vi "cic_test3.vi"() -> ()   [LabVIEW 2013]
panel:
  out "Waveform Graph out 2":i16[](graph)
  out "Waveform Graph out":dbl[](graph)
  out "Waveform Graph":dbl[](graph)
  out "# of Iterations":i32
  out "# of samples":i32
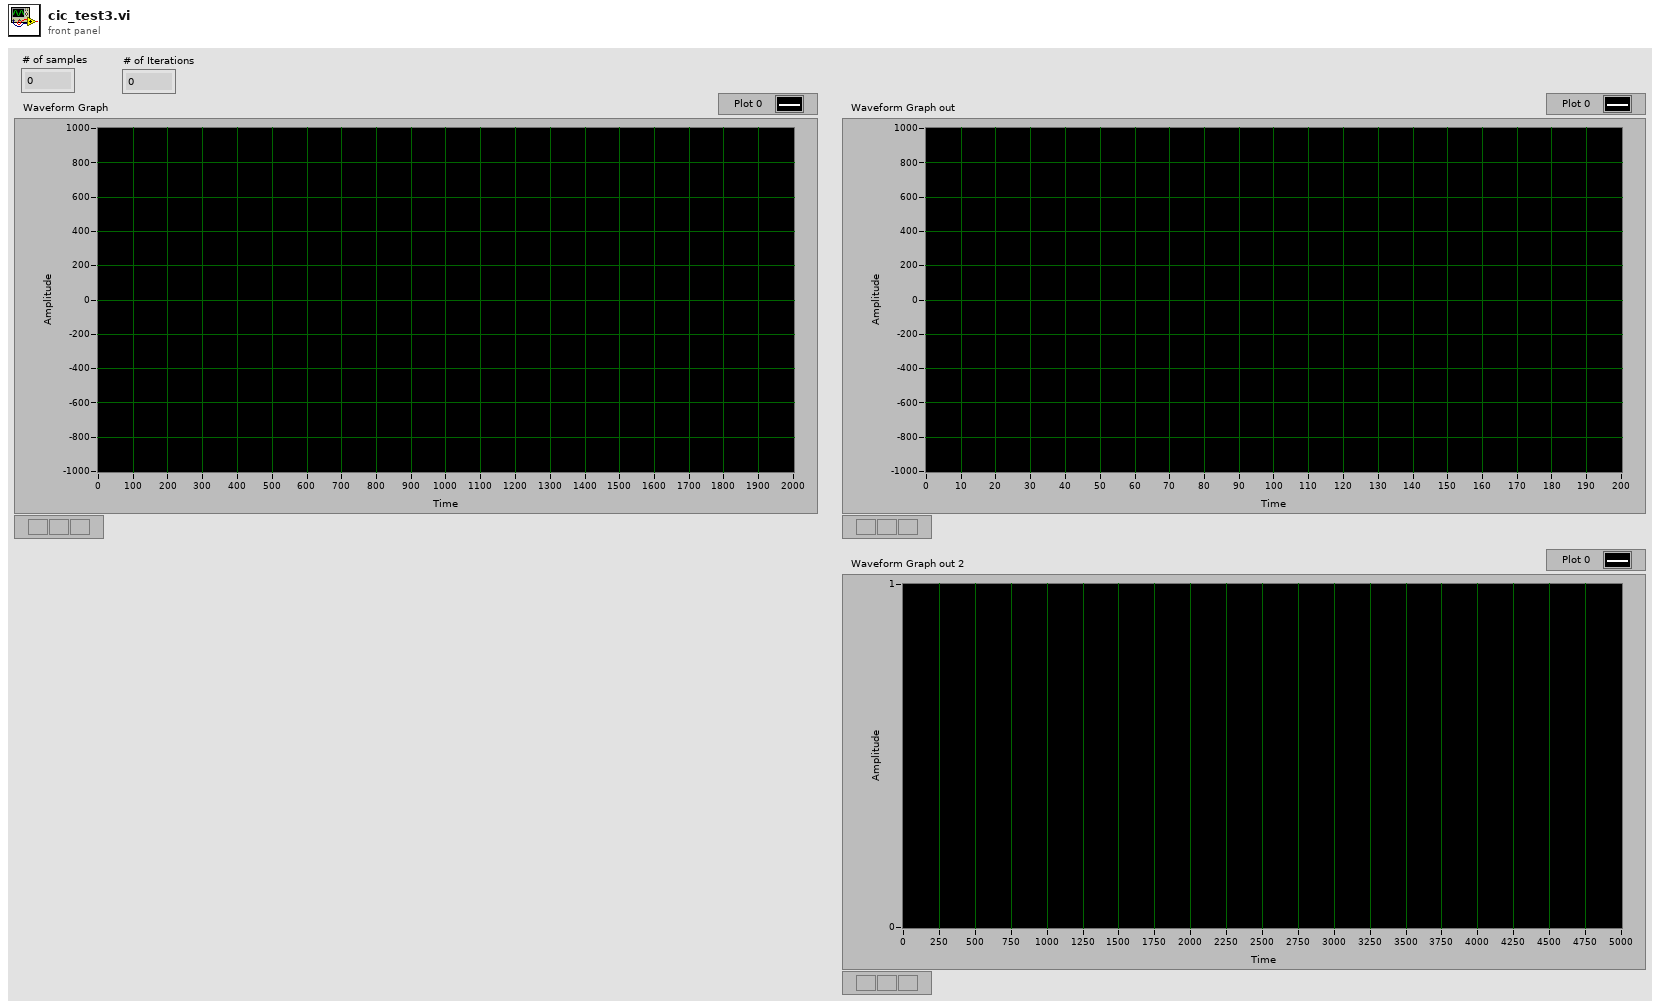
[diagram p1: front panel]
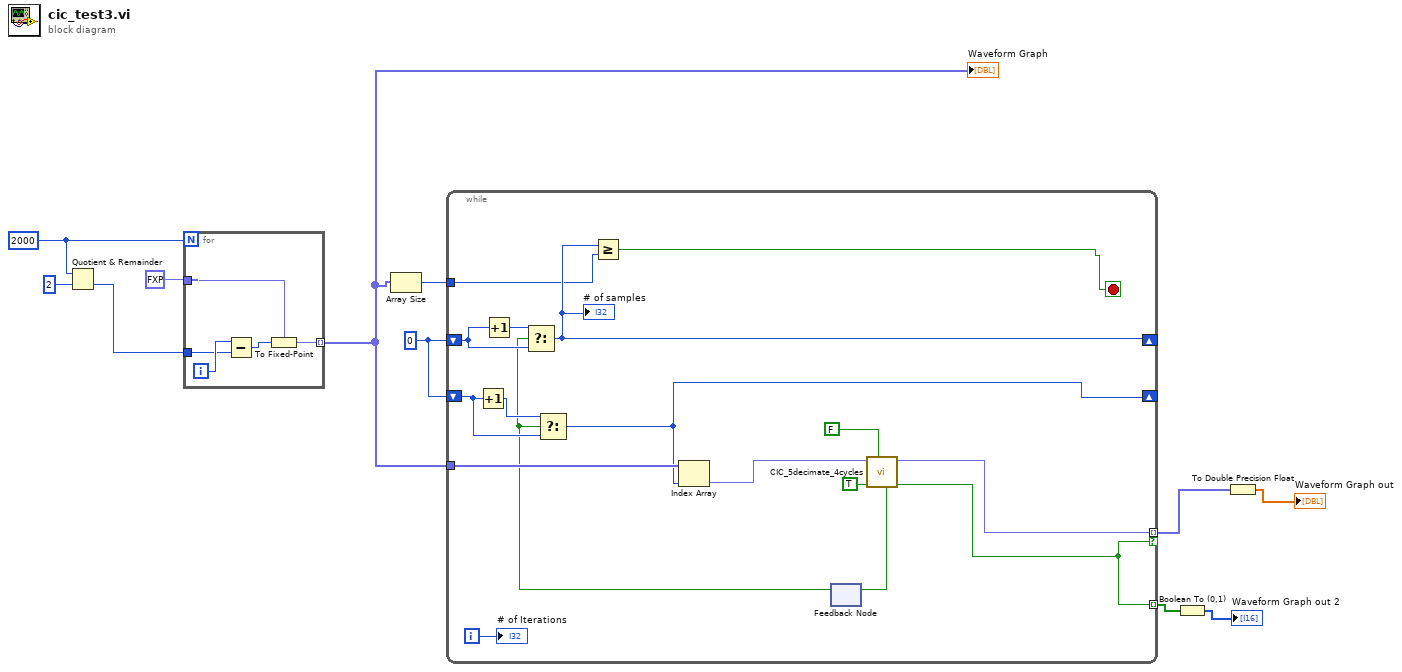
[diagram p0: block diagram]
diagram:
  w5 = 2000
  w9 = 0 ("samples")
  n1 = Quotient & Remainder(x=w5, y=2) -> (floor(x/y)=w3:i32)  [unwired: 1 out]
  n2 = for {
    N: w5 -> [_]
    tunnel: fxp<+/-,16,14> 0.0 ("fixed-point type") -> [w16]
    tunnel: [w15] -> w6 mode=indexing
    tunnel: w3 -> [w13]
    i -> [w14]
    n3 = Subtract(x=w14, y=w13) -> (x-y=w12:i32)
    n4 = To Fixed-Point(fixed-point type=w16, number=w12) -> (fixed-point=w15:fxp<+/-,16,14>)
  }
  "Waveform Graph" <- w6
  n5 = Array Size(array=w6) -> (size(s)=w10:i32)
  n6 = while {
    tunnel: w6 -> [w33]
    shift-right: [w25] -> _
    shift-left: w9 -> [w31]
    shift-right: [w28] -> _
    shift-left: w9 -> [w29]
    tunnel: [w19] -> w8 mode=indexing if=w17
    tunnel: w10 -> [w26]
    tunnel: [w17] -> w2 mode=indexing
    i -> [w24]
    stop <- w27 stop-if-true
    n7 = Increment(x=w31) -> (x+1=w32:i32)
    n8 = Increment(x=w29) -> (x+1=w30:i32)
    n9 = feedback #1() -> (w18:bool)  [unwired: 1 in]
    n10 = Select(t=w30, s=w18, f=w29) -> (s? t:f=w28:i32)
    "# of samples" <- w28
    n11 = Select(t=w32, s=w18, f=w31) -> (s? t:f=w25:i32)
    n12 = Greater Or Equal?(x=w28, y=w26) -> (x >= y?=w27:bool)
    n13 = Index Array(array=w33, index=w25) -> (element=w23:fxp<+/-,16,14>)
    n14 = call "CIC_5decimate_4cycles.vi"("reset"=FALSE, "valid in"=TRUE, "Data in"=w23) -> ("valid out"=w17:bool, "Data out"=w19:fxp<+/-,16,14>, "ready for input"=w22:bool)  [unwired: 6 in]
    n15 = feedback-in #1(w22) -> ()
    "# of Iterations" <- w24
  }
  n16 = Boolean To (0,1)(Boolean=w2) -> (0, 1=→"Waveform Graph out 2":i16[])
  n17 = To Double Precision Float(number=w8) -> (double precision float=→"Waveform Graph out":dbl[])
